vi "Insert Variable.vi"(8 "error in (no error)":errorcluster, 11 "Python Protocol in":refnum<class "Python Protocol.lvclass">) -> (0 "error out":errorcluster, 3 "Python Protocol out":refnum<class "Python Protocol.lvclass">)   [LabVIEW 2013, in "Python Protocol.lvlib" / "Python Protocol.lvclass"]
uses:
  Python Protocol.lvclass
  Python Protocol.lvclass/Python Protocol.ctl
  Read Code.vi
  Read Ring Refnum.vi
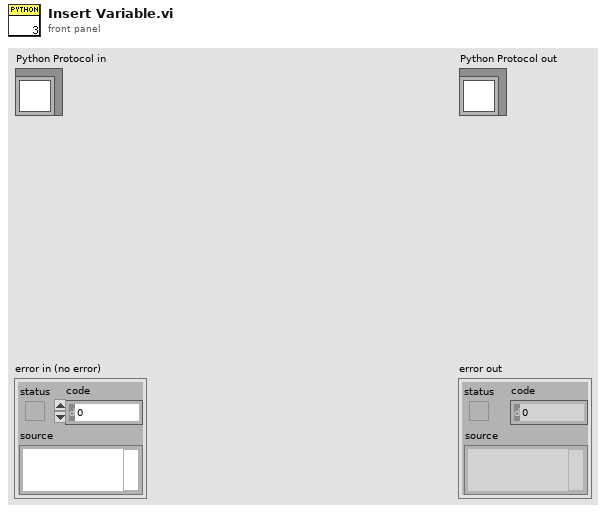
[diagram p1: front panel]
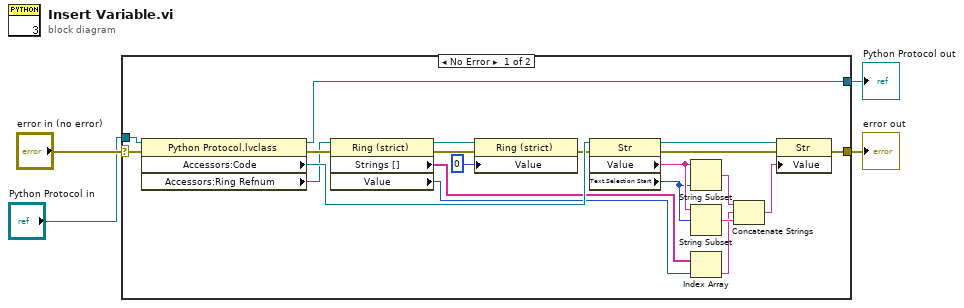
[diagram p0: block diagram]
diagram:
  n1 = case shown="No Error" "error in (no error)" {
    selector: "error in (no error)" -> [w14 w27]
    tunnel: [w15 w27] -> w3
    tunnel: [w24 w26] -> w1
    tunnel: "Python Protocol in" -> [w25 w26]
    frame No Error {
      n2 = property class="Python Protocol.lvclass"(reference=w25, error in=w14) -> (reference out=w24:refnum<class "Python Protocol.lvclass">, error out=w13:errorcluster, "Accessors:Code"=w17:refnum<vi>, "Accessors:Ring Refnum"=w12:refnum<vi>)
      n3 = property class="Ring (strict)"(reference=w12, error in=w13) -> (reference out=w8:refnum<vi>, error out=w7:errorcluster, "Strings []"=w11:string[], "Value"=w10:u16)
      n4 = property class="Ring (strict)"(reference=w8, error in=w7, "Value"=u16 0) -> (error out=w6:errorcluster)  [unwired: 1 out]
      n5 = property class="Str"(reference=w17, error in=w6) -> (reference out=w19:refnum<vi>, error out=w16:errorcluster, "Value"=w23:string, "Text.Selection Start"=w22:u32)
      n6 = String Subset(string=w23, length (rest)=w22) -> (substring=w21:string)  [unwired: 1 in]
      n7 = String Subset(string=w23, offset (0)=w22) -> (substring=w20:string)  [unwired: 1 in]
      n8 = Index Array(array=w11, index=w10) -> (element=w9:string)
      n9 = Concatenate Strings(w21, w9, w20) -> (w18:string)
      n10 = property class="Str"(reference=w19, error in=w16, "Value"=w18) -> (error out=w15:errorcluster)  [unwired: 1 out]
    }
    frame Error {
    }
  }
  "error out" <- w3
  "Python Protocol out" <- w1
